vi "Mem Compilation Tester.vi"() -> ()   [LabVIEW 2013]
uses:
  <vilib>/Platform/TimedLoop/XDataNode/timing_clust.ctl
  <vilib>/Platform/TimedLoop/XDataNode/nitl_modes.ctl
  <vilib>/Platform/TimedLoop/XDataNode/wakeup.ctl
  <vilib>/rvi/Emulation/niFpgaSctlEmulationGetInTimedLoop.vi
  <vilib>/rvi/Emulation/niFpgaEmulationReportErrorSimple.vi
  <vilib>/rvi/Emulation/niFpgaGetClockAttributes.vi
  <vilib>/rvi/Emulation/niFpgaCriticalErrorInLSC.vi
  <vilib>/rvi/FIFO/Fifo_Resource/nirvififoEmulationWriteFpgaImpl.vi
  <vilib>/rvi/DataTransferAndStorage/Container/Common/niFpgaContainerGetUniqueNameForEmu.vi
  <vilib>/Platform/TimedLoop/XDataNode/XDataNode.xnode
  <vilib>/rvi/DataTransferAndStorage/Container/XNode/niFpgaContainer.xnode
  <vilib>/rvi/FIFO/Fifo_Resource/nirvififoEmulationWrite.vi
  <vilib>/rvi/FIFO/Fifo_Resource/nirvififoEmulationRead.vi
  <vilib>/Platform/TimedLoop/XDataNode/XDNodeRunTimeDep.lvlib
panel:
  out "Timed Out?":bool
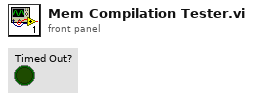
[diagram p1: front panel]
types:
  T1 = typedef "XDNodeRunTimeDep.lvlib/timing_clust.ctl" = cluster{"Expected End [f-1]":u64, "Actual End [f-1]":u64, "Finished Late? [f-1]":bool, "Expected End [i-1]":u64, "Actual End [i-1]":u64, "Finished Late? [i-1]":bool, "Expected Start [i]":u64, "Actual Start [i]":u64, "Expected Start [f]":u64, "Actual Start [f]":u64, "Source Name":string, "Structure Name":string, "Period":i64, "Deadline":i64, "Offset":i64, "Start":i64, "Priority":i32, "Timeout":i32, "Mode":T2, "Wakeup Reason":T3, "Error":errorcluster, "Source Type":string, "Secondary Source Type":string, "Global End Time":u64, "Global Start Time":u64, "Frame Duration":u64, "Iteration Duration":u64, "Assigned CPU":i32, "I/O Scan Engine Mode":u32}
  T2 = typedef "XDNodeRunTimeDep.lvlib/nitl_modes.ctl" = enum32{"No Change", "Process missed periods, maintain original phase", "Discard missed periods, maintain original phase", "Process missed periods, ignore original phase", "Discard missed periods, ignore original phase"}
  T3 = typedef "XDNodeRunTimeDep.lvlib/wakeup.ctl" = enum32{"Normal", "Aborted", "Asynchronous wakeup", "Timing source error", "Timed loop error", "Timeout"}
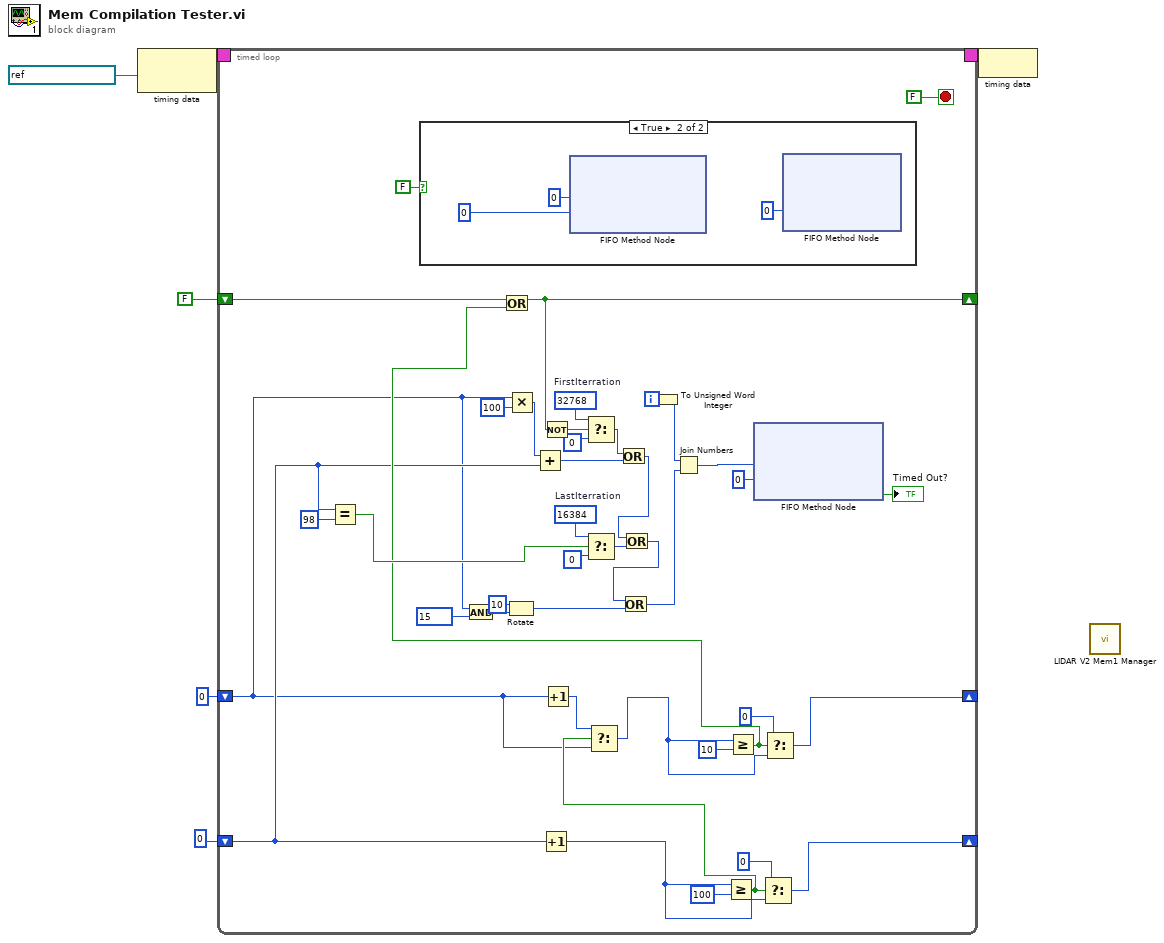
[diagram p0: block diagram]
diagram:
  n1 = node-c288(refnum<k21> "100 MHz Clock" ("Source Name")) -> (w3:T1)
  n2 = timed-loop {
    shift-right: [w7] -> _
    shift-left: u8 0 -> [w8]
    shift-right: [w9] -> _
    shift-left: u16 0 -> [w10]
    shift-right: [w12] -> _
    shift-left: FALSE -> [w14]
    timing: w3 -> [_]
    timing-out: [_] -> w2
    i -> [w19]
    stop <- FALSE stop-if-true
    w37 = u16 16384  # LastIterration
    w34 = u16 32768  # FirstIterration
    n3 = Equal?(x=w10, y=u16 98) -> (x = y?=w20:bool)
    n4 = case shown="True" FALSE {
      frame False {
      }
      frame True {
        n5 = xnode ("FIFO Method Node")("Element"=u32 0, "Timeout"=0) -> ()  [unwired: 1 in, 2 out]
        n6 = xnode ("FIFO Method Node")("Timeout"=0) -> ()  [unwired: 1 in, 3 out]
      }
    }
    n7 = And(x=w8, y=u16 15) -> (x .and. y?=w41:u16)
    n8 = Rotate(1:w41, 2:i16 10 ("y")) -> (0:w43:u16)
    n9 = Multiply(x=w8, y=u16 100) -> (x*y=w31:u16)
    n10 = Add(x=w31, y=w10) -> (x+y=w32:u16)
    n11 = Increment(x=w10) -> (x+1=w22:u16)
    n12 = Increment(x=w8) -> (x+1=w25:u8)
    n13 = Select(t=w37, s=w20, f=u16 0 ("x")) -> (s? t:f=w38:u16)
    n14 = To Unsigned Word Integer(number=w19) -> (unsigned 16bit integer=w16:u16)
    n15 = Greater Or Equal?(x=w22, y=u8 100) -> (x >= y?=w17:bool)
    n16 = Select(t=w25, s=w17, f=w8) -> (s? t:f=w26:u8)
    n17 = Greater Or Equal?(x=w26, y=u8 10) -> (x >= y?=w13:bool)
    n18 = Or(x=w14, y=w13) -> (x .or. y?=w12:bool)
    n19 = Not(x=w12) -> (.not. x?=w11:bool)
    n20 = Select(t=w34, s=w11, f=u16 0 ("x")) -> (s? t:f=w33:u16)
    n21 = Or(x=w33, y=w32) -> (x .or. y?=w39:u16)
    n22 = Or(x=w39, y=w38) -> (x .or. y?=w44:u16)
    n23 = Or(x=w44, y=w43) -> (x .or. y?=w45:u16)
    n24 = Join Numbers(hi=w16, lo=w45) -> ((hi.lo)=w29:u32)
    n25 = xnode ("FIFO Method Node")("Element"=w29, "Timeout"=0) -> ("Timed Out?"=→"Timed Out?":bool)  [unwired: 1 in, 1 out]
    n26 = Select(t=u8 0, s=w17, f=w22) -> (s? t:f=w9:u16)
    n27 = Select(t=u8 0, s=w13, f=w26) -> (s? t:f=w7:u8)
  }
  n28 = node-c288(w2) -> ()
  n29 = call "LIDAR V2 Mem1 Manager.vi"() -> ()  [unwired: 12 in]
